vi "CompressAndUpdate(ScopeTraceBinary).vi"(6 "wfm info":T1, 7 "force CVT update (false)":bool, 8 "error in":errorcluster, 9 "precision (12)":i16=12, 10 "wfm":i16[](array[numeric]), 11 "command or variable name":string) -> (0 "error out":errorcluster, 3 "Trace String":string)   [LabVIEW 2011]
panel:
  out "x-y":u32(graph)
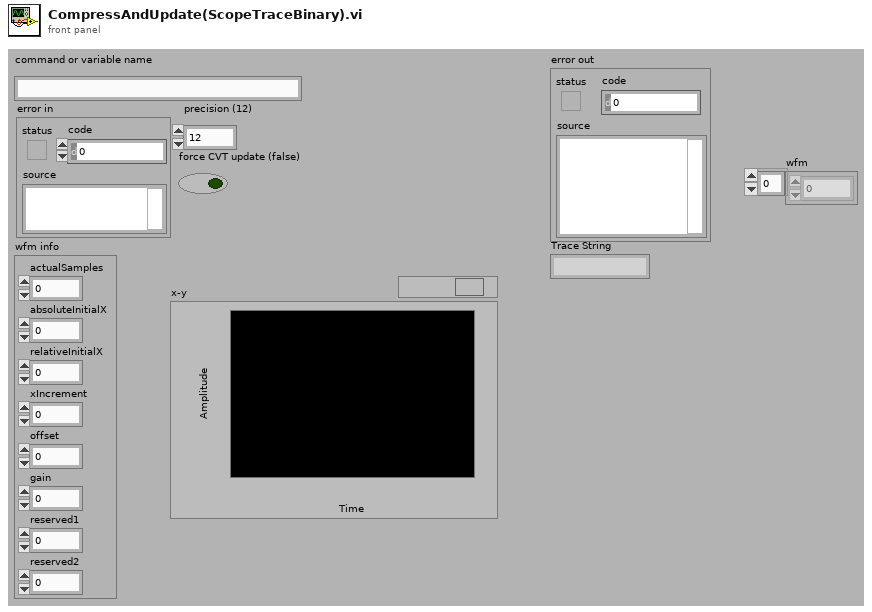
[diagram p1: front panel]
types:
  T1 = cluster{"actualSamples":i32, "absoluteInitialX":dbl, "relativeInitialX":dbl, "xIncrement":dbl, "offset":dbl, "gain":dbl, "reserved1":dbl, "reserved2":dbl}
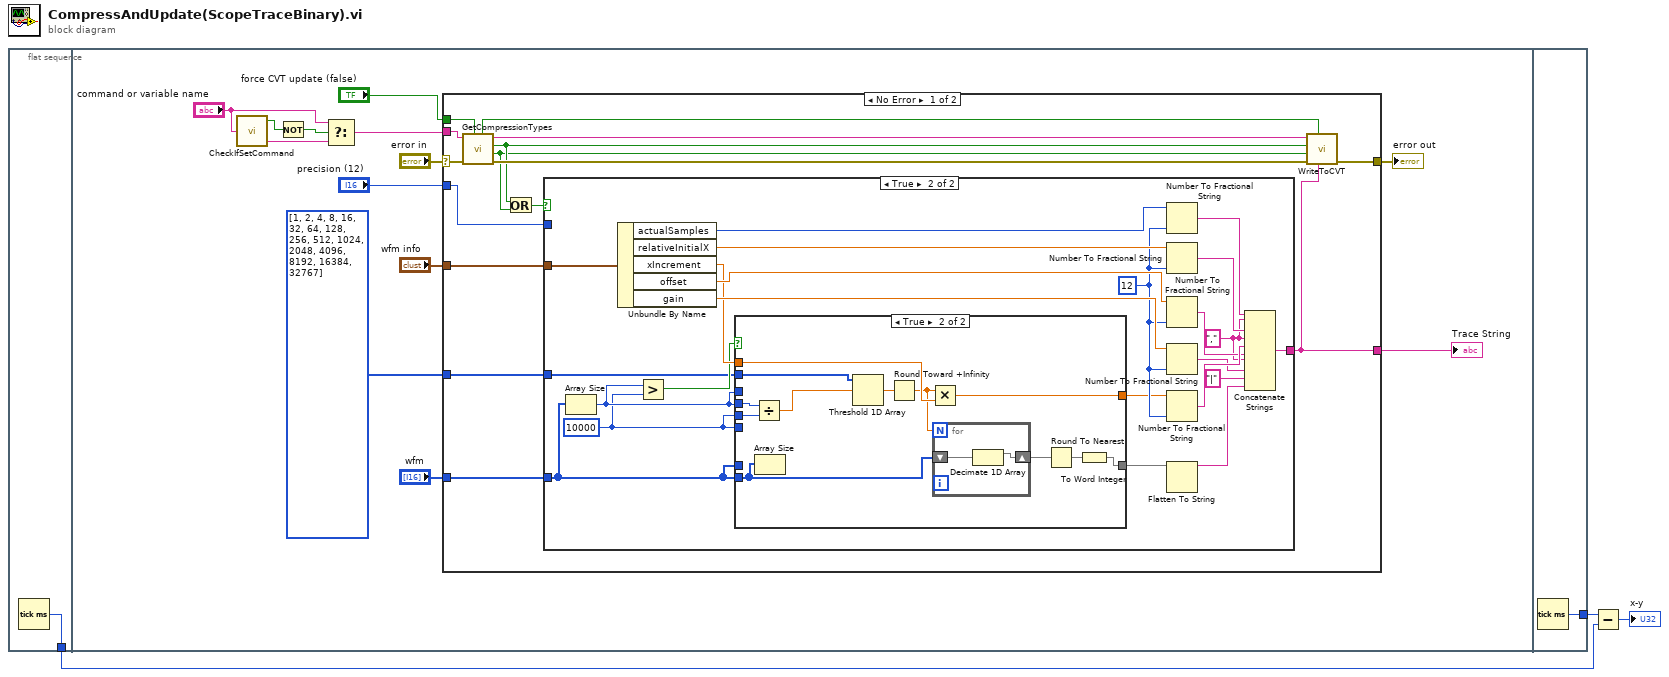
[diagram p0: block diagram]
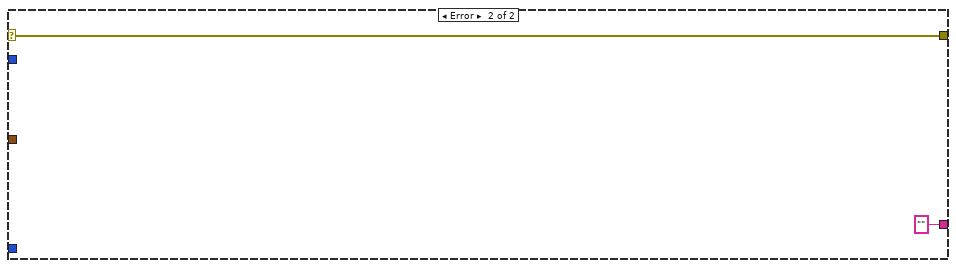
[diagram p4: hidden frame]
diagram:
  n1 = flat-sequence {
    tunnel: [w4] -> w2
    tunnel: [w74] -> w3
    frame #0 {
      n2 = Tick Count (ms)() -> (millisecond timer value=w4:u32)
    }
    frame #1 {
      n3 = call "CheckIfSetCommand.vi"("Command"="command or variable name") -> ("setCommand?"=w14:bool, "variable"=w12:string)  [unwired: 1 out]
      n4 = Not(x=w14) -> (.not. x?=w15:bool)
      n5 = Select(t="command or variable name", s=w15, f=w12) -> (s? t:f=w11:string)
      n6 = case shown="No Error" "error in" {
        selector: "error in" -> [w32 w73]
        tunnel: [w26 w73] -> w17
        tunnel: w11 -> [w27 _]
        tunnel: "wfm" -> [w31 _]
        tunnel: "precision (12)" -> [w30 _]
        tunnel: "force CVT update (false)" -> [w25 _]
        tunnel: [w20 ""] -> w7
        tunnel: "wfm info" -> [w19 _]
        tunnel: i16[] [1, 2, 4, 8, 16, 32, 64, 128, 256, 512, 1024, 2048, 4096, 8192, 16384, 32767] -> [w18 _]
        frame No Error {
          n7 = call "GetCompressionTypes.vi"("force CVT update"=w25, "error in"=w32, "variable"=w27) -> ("error out"=w28:errorcluster, "non compressed"=w21:bool, "compressed"=w22:bool, "variable out"=w23:string, "force CVT update out"=w24:bool)  [unwired: 4 in]
          n8 = Or(x=w22, y=w21) -> (x .or. y?=w29:bool)
          n9 = case shown="True" w29 {
            tunnel: w31 -> [_ w37]
            tunnel: w30 -> [_ _]
            tunnel: [_ w50] -> w20
            tunnel: w19 -> [_ w55]
            tunnel: w18 -> [_ w33]
            frame False {
            }
            frame True {
              w35 = 10000 ("y")
              w41 = i16 12 ("precision (6)")
              w44 = "," ("string")
              n10 = Array Size(array=w37) -> (size(s)=w36:i32)
              n11 = Unbundle By Name(w55) -> ("actualSamples"=w54:i32, "relativeInitialX"=w53:dbl, "xIncrement"=w40:dbl, "offset"=w52:dbl, "gain"=w51:dbl)
              n12 = Greater?(x=w36, y=w35) -> (0:w34:bool)
              n13 = case shown="True" w34 {
                tunnel: w37 -> [w56 _]
                tunnel: w40 -> [w57 w65]
                tunnel: [w57 w64] -> w39
                tunnel: [w56 w68] -> w38
                tunnel: w36 -> [_ _]
                tunnel: w35 -> [_ _]
                tunnel: w37 -> [_ w63]
                tunnel: w36 -> [_ w67]
                tunnel: w35 -> [_ w66]
                tunnel: w33 -> [_ w60]
                frame False {
                }
                frame True {
                  n14 = Divide(x=w67, y=w66) -> (x/y=w61:dbl)
                  n15 = Array Size(array=w63) -> ()  [unwired: 1 out]
                  n16 = Threshold 1D Array(2:w61, 3:w60) -> (0:w59:dbl)  [unwired: 1 in]
                  n17 = Round Toward +Infinity(x=w59) -> (ceil(x): smallest int >= x=w58:dbl)
                  n18 = Multiply(x=w58, y=w65) -> (x*y=w64:dbl)
                  n19 = for {
                    N: w58 -> [_]
                    shift-right: [w70] -> w62
                    shift-left: w63 -> [w71]
                    n20 = Decimate 1D Array(w71) -> (w70:i16[])  [unwired: 1 out]
                  }
                  n21 = Round To Nearest(number=w62) -> (nearest integer value=w69:i16[])
                  n22 = To Word Integer(number=w69) -> (16bit integer=w68:i16[])
                }
              }
              n23 = Number To Fractional String(number=w54, precision (6)=w41) -> (F-format string=w49:string)  [unwired: 2 in]
              n24 = Number To Fractional String(number=w53, precision (6)=w41) -> (F-format string=w48:string)  [unwired: 2 in]
              n25 = Number To Fractional String(number=w52, precision (6)=w41) -> (F-format string=w46:string)  [unwired: 2 in]
              n26 = Number To Fractional String(number=w51, precision (6)=w41) -> (F-format string=w45:string)  [unwired: 2 in]
              n27 = Number To Fractional String(number=w39, precision (6)=w41) -> (F-format string=w47:string)  [unwired: 2 in]
              n28 = Flatten To String(anything=w38) -> (data string=w43:string)  [unwired: 3 in, 2 out]
              n29 = Concatenate Strings(w49, w44, w48, w44, w47, w46, w44, w45, "|" ("string"), w43) -> (w50:string)
            }
          }
          n30 = call "WriteToCVT.vi"("compressed string"=w20, "force CVT update"=w24, "error in"=w28, "non compressed"=w21, "compressed"=w22, "variable"=w23) -> ("error out"=w26:errorcluster)  [unwired: 5 in]
        }
        frame Error {
        }
      }
      "error out" <- w17
      "Trace String" <- w7
    }
    frame #2 {
      n31 = Tick Count (ms)() -> (millisecond timer value=w74:u32)
    }
  }
  n32 = Subtract(x=w3, y=w2) -> (x-y=→"x-y":u32)
